vi "build waypoint url.vi"(8 "error in (no error)":errorcluster, 11 "System":string) -> (0 "error out":errorcluster, 3 "url":string)   [LabVIEW 2024, in "GUI.lvlib" / "Functions.lvlib"]
uses:
  Functions.lvlib
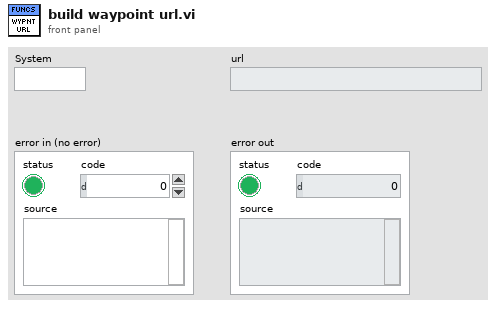
[diagram p1: front panel]
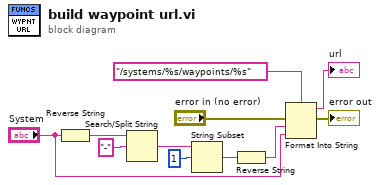
[diagram p0: block diagram]
diagram:
  n1 = Reverse String(1:"System") -> (0:w8:string)
  n2 = Search/Split String(string=w8, search string/char (-)="-") -> (match + rest of string=w3:string)  [unwired: 1 in, 2 out]
  n3 = String Subset(string=w3, offset (0)=1) -> (substring=w2:string)  [unwired: 1 in]
  n4 = Reverse String(1:w2) -> (0:w1:string)
  n5 = Format Into String(format string="/systems/%s/waypoints/%s", error in="error in (no error)", w1, "System") -> (resulting string=→"url":string, error out=→"error out":errorcluster)  [unwired: 1 in]
